vi "new_FGGA_read.vi"() -> ()   [LabVIEW 2014]
uses:
  <vilib>/Utility/RT CPU Load.ctl
  <vilib>/Instr/_visa.llb/VISA Set IO Buffer Mask.ctl
  <vilib>/Instr/_visa.llb/VISA Flush IO Buffer Mask.ctl
  <vilib>/Platform/TimedLoop/XDataNode/timing_clust.ctl
  <vilib>/Platform/TimedLoop/XDataNode/nitl_modes.ctl
  <vilib>/Platform/TimedLoop/XDataNode/wakeup.ctl
  <vilib>/Instr/_visa.llb/VISA Configure Serial Port (Instr).vi
  <vilib>/platform/TimedLoop/XDataNode/XDataNode.xnode
  <vilib>/Platform/TimedLoop/XDataNode/XDNodeRunTimeDep.lvlib
  <vilib>/NI_Real-Time Target Support.lvlib
panel:
  out "Waveform Chart":dbl(graph)
  out "CPU loads":T1[](array[typedef]) {"ISR (%)" format="%#.2f"; "Idle (%)" format="%#.2f"; "Background (%)" format="%#.2f"; "Normal (%)" format="%#.2f"; "Above Normal (%)" format="%#.2f"; "High (%)" format="%#.2g"; "Timed Structures (%)" format="%#.2g"; "Time Critical (%)" format="%#.2g"; "Total (%)" format="%#.2g"}
  out "Queue Out":string
  in  "VISA resource name":refnum<visa-resource-name>="ASRL7::INSTR"
  in  "timeout (10sec)":u32=1500
  out "error out":errorcluster
  out "String":string
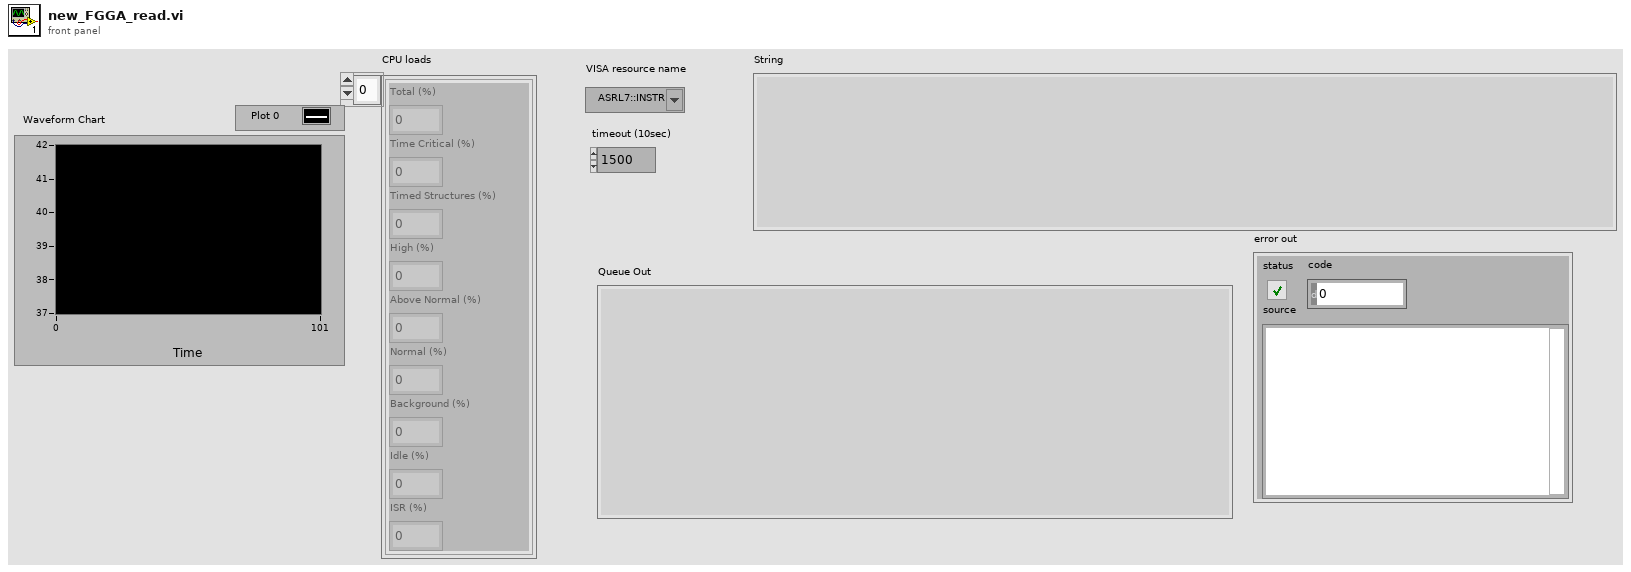
[diagram p1: front panel]
types:
  T1 = typedef "NI_Real-Time Target Support.lvlib/RT CPU Load.ctl" = cluster{"Total (%)":dbl, "Time Critical (%)":dbl, "Timed Structures (%)":dbl, "High (%)":dbl, "Above Normal (%)":dbl, "Normal (%)":dbl, "Background (%)":dbl, "Idle (%)":dbl, "ISR (%)":dbl}
  T2 = typedef "VISA Flush IO Buffer Mask.ctl" = u16
  T3 = typedef "VISA Set IO Buffer Mask.ctl" = u16
  T4 = typedef "XDNodeRunTimeDep.lvlib/timing_clust.ctl" = cluster{"Expected End [f-1]":u64, "Actual End [f-1]":u64, "Finished Late? [f-1]":bool, "Expected End [i-1]":u64, "Actual End [i-1]":u64, "Finished Late? [i-1]":bool, "Expected Start [i]":u64, "Actual Start [i]":u64, "Expected Start [f]":u64, "Actual Start [f]":u64, "Source Name":string, "Structure Name":string, "Period":i64, "Deadline":i64, "Offset":i64, "Start":i64, "Priority":i32, "Timeout":i32, "Mode":T5, "Wakeup Reason":T6, "Error":errorcluster, "Source Type":string, "Secondary Source Type":string, "Global End Time":u64, "Global Start Time":u64, "Frame Duration":u64, "Iteration Duration":u64, "Assigned CPU":i32, "I/O Scan Engine Mode":u32}
  T5 = typedef "XDNodeRunTimeDep.lvlib/nitl_modes.ctl" = enum32{"No Change", "Process missed periods, maintain original phase", "Discard missed periods, maintain original phase", "Process missed periods, ignore original phase", "Discard missed periods, ignore original phase"}
  T6 = typedef "XDNodeRunTimeDep.lvlib/wakeup.ctl" = enum32{"Normal", "Aborted", "Asynchronous wakeup", "Timing source error", "Timed loop error", "Timeout"}
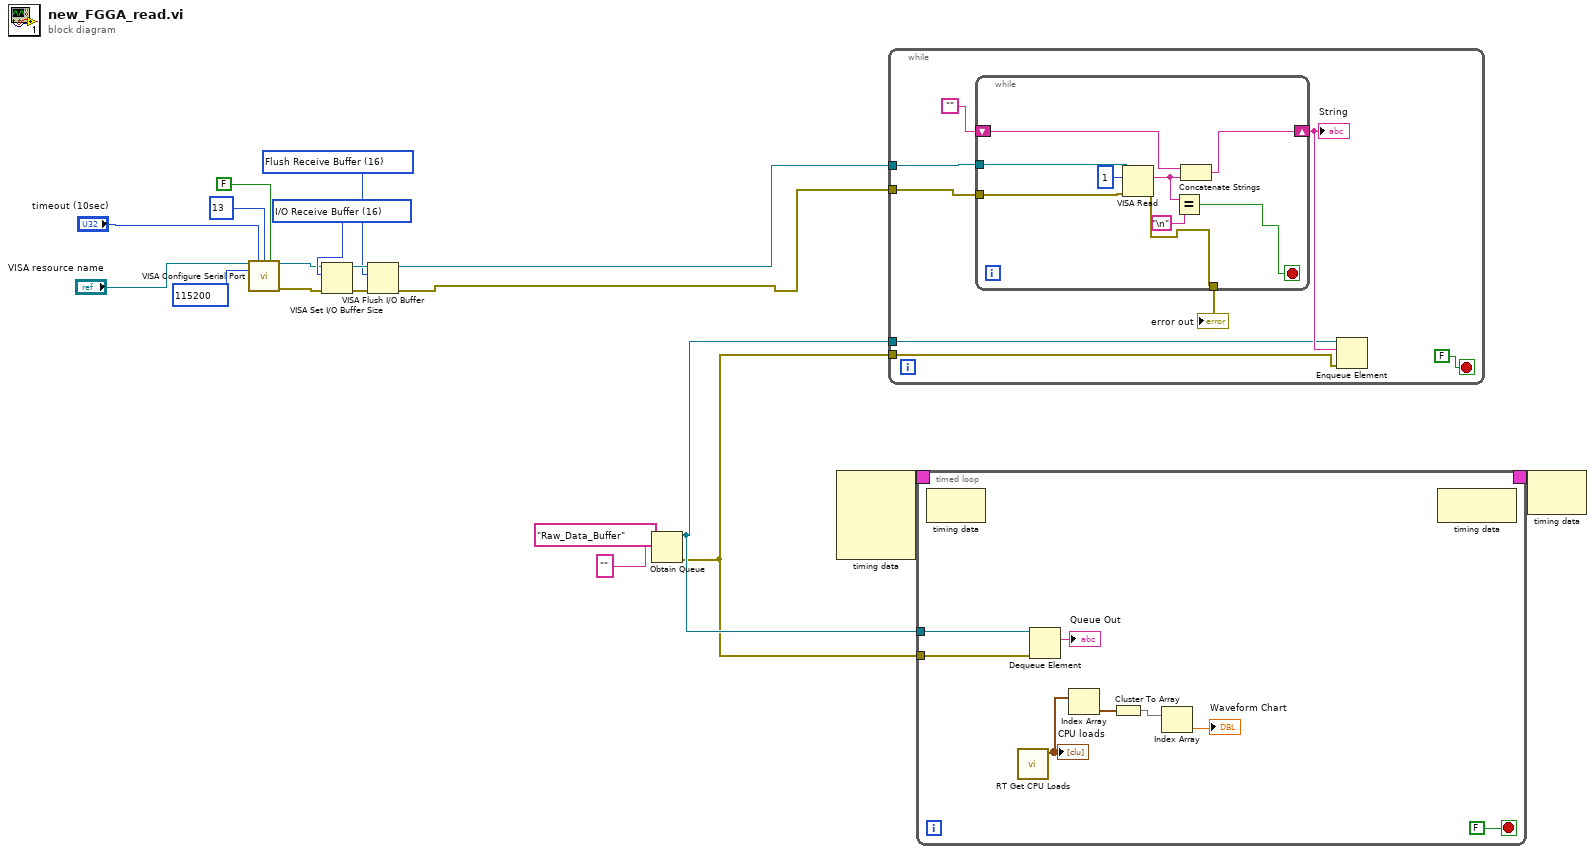
[diagram p0: block diagram]
diagram:
  w12 = T2 16 items=["Flush Receive Buffer"=16, "Write Transmit Buffer to Device"=32, "Flush Receive Buffer (No I/O)"=64, "Flush Transmit Buffer"=128] ("Mask")
  w13 = T3 16 items=["I/O Receive Buffer"=16, "I/O Transmit Buffer"=32, "I/O Receive and Transmit Buffer"=48] ("Mask")
  n1 = call-poly "VISA Configure Serial Port"("VISA resource name"="VISA resource name", "timeout (10sec)"="timeout (10sec)", "termination char\n(0xA = '\\n' = LF)"=u8 13 ("termination char\n(0xA = '\\n' = LF)"), "Enable Termination\nChar (T)"=FALSE ("Enable Termination\nChar (T)"), "baud rate (9600)"=u32 115200) -> ("VISA resource name out"=w11:refnum<visa-resource-name>, "error out"=w10:errorcluster)  [unwired: 9 in]
  n2 = VISA Set I/O Buffer Size(VISA resource name=w11, mask (16)=w13, error in (no error)=w10) -> (VISA resource name out=w14:refnum<visa-resource-name>, error out=w15:errorcluster)  [unwired: 1 in]
  n3 = VISA Flush I/O Buffer(VISA resource name=w14, mask (16)=w12, error in (no error)=w15) -> (VISA resource name out=w8:refnum<visa-resource-name>, error out=w7:errorcluster)
  n4 = Obtain Queue(name (unnamed)="Raw_Data_Buffer", element data type="") -> (queue out=w2:refnum<queue>, error out=w1:errorcluster)  [unwired: 3 in, 1 out]
  n5 = node-c288() -> (w4:T4)  [unwired: 4 in]
  n6 = while {
    tunnel: w8 -> [w25]
    tunnel: w7 -> [w24]
    tunnel: w2 -> [w21]
    tunnel: w1 -> [w20]
    stop <- FALSE stop-if-true
    n7 = while {
      tunnel: w25 -> [w36]
      shift-right: [w33] -> w22
      shift-left: "" -> [w34]
      tunnel: w24 -> [w30]
      tunnel: [w29] -> w26
      stop <- w28 stop-if-true
      n8 = VISA Read(VISA resource name=w36, byte count=u32 1, error in (no error)=w30) -> (read buffer=w32:string, error out=w29:errorcluster)  [unwired: 2 out]
      n9 = Equal?(x=w32, y="\n") -> (x = y?=w28:bool)
      n10 = Concatenate Strings(w34, w32) -> (w33:string)
    }
    "String" <- w22
    "error out" <- w26
    n11 = Enqueue Element(queue=w21, element=w22, error in (no error)=w20) -> ()  [unwired: 1 in, 3 out]
  }
  n12 = timed-loop {
    timing: w4 -> [_]
    timing-out: [_] -> w3
    tunnel: w2 -> [w44]
    tunnel: w1 -> [w43]
    stop <- FALSE stop-if-true
    n13 = node-c288() -> ()  [unwired: 1 in, 1 out]
    n14 = call <vilib>:"RT Get CPU Loads.vi"() -> ("CPU loads"=w38:T1[])  [unwired: 10 in, 1 out]
    "CPU loads" <- w38
    n15 = Dequeue Element(queue=w44, error in (no error)=w43) -> (element=→"Queue Out":string)  [unwired: 1 in, 3 out]
    n16 = Index Array(array=w38) -> (element=w39:T1)  [unwired: 1 in]
    n17 = Cluster To Array(cluster=w39) -> (array=w40:dbl[])
    n18 = Index Array(array=w40) -> (element=→"Waveform Chart":dbl)  [unwired: 1 in]
    n19 = node-c288() -> ()  [unwired: 1 in, 1 out]
  }
  n20 = node-c288(w3) -> ()  [unwired: 1 out]
